vi "Single_to_Double.vi"(11 "DECIMAL VALUE":u16[](array[numeric])) -> (2 "Array 2":u16[](array[numeric]), 3 "Array":i16[](array[numeric]))   [LabVIEW 2017]
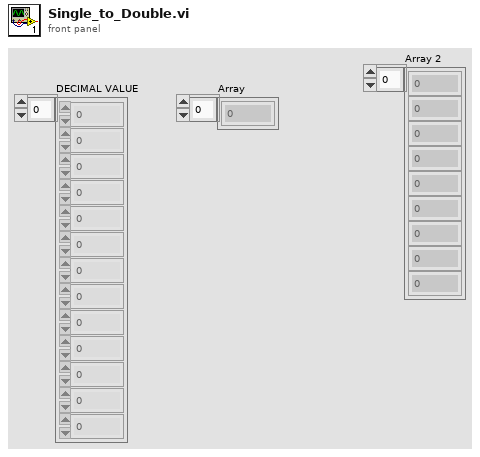
[diagram p1: front panel]
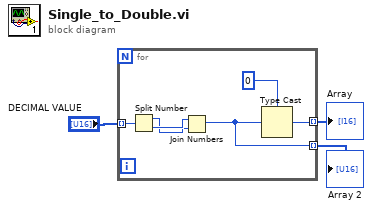
[diagram p0: block diagram]
diagram:
  n1 = for {
    tunnel: [w5] -> w3 mode=indexing
    tunnel: "DECIMAL VALUE" -> [w6] mode=indexing
    tunnel: [w4] -> w1 mode=indexing
    n2 = Split Number(x=w6) -> (hi(x)=w7:u8, lo(x)=w8:u8)
    n3 = Join Numbers(hi=w8, lo=w7) -> ((hi.lo)=w4:u16)
    n4 = Type Cast(type=i16 0, x=w4) -> (*(type *) &x=w5:i16)
  }
  "Array" <- w3
  "Array 2" <- w1
